vi "SpecAn Marker Peak Read.vi"(0 "VISA In":refnum<visa-resource-name>="N9030A", 5 "Error In":errorcluster={"status"=FALSE, "code"=1073676294, "source"="VISA Read in RS232 Send.vi->Utility Com Write.vi->CG UUT Attenuator Set.vi->CG RF Cal_00.vi"}, 7 "Active Marker":i32(ring)=1 items=["Marker1"=1, "Marker2"=2, "Marker3"=3, "Marker4"=4, "Marker5"=5, "Marker6"=6, "Marker7"=7, "Marker8"=8, "Marker9"=9, "Marker10"=10, "Marker11"=11, "Marker12"=12]) -> (10 "Freq (Hz)":dbl=599400000.0 format="%#_6p", 12 "Amplitude (dBm)":dbl=-83.196 format="%#_6p", 14 "VISA Out":refnum<visa-resource-name>="N9030A", 19 "Error Out":errorcluster={"status"=FALSE, "code"=1073676294, "source"="VISA Read in RS232 Send.vi->Utility Com Write.vi->CG UUT Attenuator Set.vi->CG RF Cal_00.vi"})   [LabVIEW 2015]
uses:
  Controls/FGV Action SpecAn Model.ctl
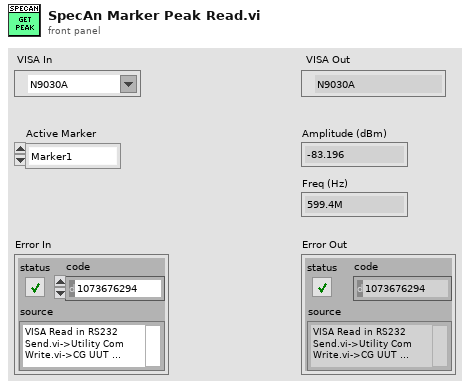
[diagram p1: front panel]
types:
  T1 = typedef "FGV Action SpecAn Model.ctl" = enum16{"Get", "Set"}
  T2 = typedef "SpecAn Model.ctl" = enum16{"E4440", "N9030"}
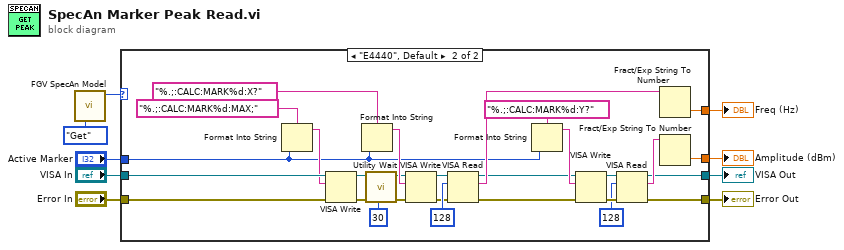
[diagram p0: block diagram]
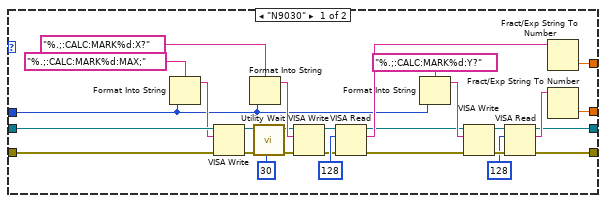
[diagram p2: hidden frame]
diagram:
  n1 = call "FGV SpecAn Model.vi"("Action"=FGV_Action_SpecAn_Model."Get") -> ("SA Model"=w1:T2)  [unwired: 6 in, 1 out]
  n2 = case shown="\"E4440\", Default" w1 {
    tunnel: "VISA In" -> [w34 w61]
    tunnel: "Error In" -> [w33 w60]
    tunnel: [w32 w59] -> w7
    tunnel: [w23 w50] -> w6
    tunnel: "Active Marker" -> [w16 w43]
    tunnel: [w14 w41] -> w4
    tunnel: [w13 w40] -> w3
    frame "N9030" {
      n3 = Format Into String(format string="%.;:CALC:MARK%d:MAX;" ("multi-line string"), w16) -> (resulting string=w31:string)  [unwired: 2 in, 1 out]
      n4 = VISA Write(VISA resource name=w34, write buffer=w31, error in (no error)=w33) -> (VISA resource name out=w28:refnum<visa-resource-name>, error out=w35:errorcluster)  [unwired: 1 out]
      n5 = Format Into String(format string="%.;:CALC:MARK%d:X?" ("multi-line string"), w16) -> (resulting string=w30:string)  [unwired: 2 in, 1 out]
      n6 = call "Utility Wait.vi"("Error In"=w35, "Wait (ms)"=u32 30) -> ("Error Out"=w29:errorcluster)  [unwired: 17 in]
      n7 = VISA Write(VISA resource name=w28, write buffer=w30, error in (no error)=w29) -> (VISA resource name out=w25:refnum<visa-resource-name>, error out=w24:errorcluster)  [unwired: 1 out]
      n8 = VISA Read(VISA resource name=w25, byte count=u32 128, error in (no error)=w24) -> (VISA resource name out=w12:refnum<visa-resource-name>, read buffer=w27:string, error out=w11:errorcluster)  [unwired: 1 out]
      n9 = Format Into String(format string="%.;:CALC:MARK%d:Y?", w16) -> (resulting string=w17:string)  [unwired: 2 in, 1 out]
      n10 = VISA Write(VISA resource name=w12, write buffer=w17, error in (no error)=w11) -> (VISA resource name out=w19:refnum<visa-resource-name>, error out=w20:errorcluster)  [unwired: 1 out]
      n11 = VISA Read(VISA resource name=w19, byte count=u32 128, error in (no error)=w20) -> (VISA resource name out=w14:refnum<visa-resource-name>, read buffer=w15:string, error out=w13:errorcluster)  [unwired: 1 out]
      n12 = Fract/Exp String To Number(string=w27) -> (number=w23:dbl)  [unwired: 3 in, 1 out]
      n13 = Fract/Exp String To Number(string=w15) -> (number=w32:dbl)  [unwired: 3 in, 1 out]
    }
    frame "E4440", Default {
      n14 = Format Into String(format string="%.;:CALC:MARK%d:MAX;" ("multi-line string"), w43) -> (resulting string=w58:string)  [unwired: 2 in, 1 out]
      n15 = VISA Write(VISA resource name=w61, write buffer=w58, error in (no error)=w60) -> (VISA resource name out=w55:refnum<visa-resource-name>, error out=w62:errorcluster)  [unwired: 1 out]
      n16 = Format Into String(format string="%.;:CALC:MARK%d:X?" ("multi-line string"), w43) -> (resulting string=w57:string)  [unwired: 2 in, 1 out]
      n17 = call "Utility Wait.vi"("Error In"=w62, "Wait (ms)"=u32 30) -> ("Error Out"=w56:errorcluster)  [unwired: 17 in]
      n18 = VISA Write(VISA resource name=w55, write buffer=w57, error in (no error)=w56) -> (VISA resource name out=w52:refnum<visa-resource-name>, error out=w51:errorcluster)  [unwired: 1 out]
      n19 = VISA Read(VISA resource name=w52, byte count=u32 128, error in (no error)=w51) -> (VISA resource name out=w39:refnum<visa-resource-name>, read buffer=w54:string, error out=w38:errorcluster)  [unwired: 1 out]
      n20 = Format Into String(format string="%.;:CALC:MARK%d:Y?", w43) -> (resulting string=w44:string)  [unwired: 2 in, 1 out]
      n21 = VISA Write(VISA resource name=w39, write buffer=w44, error in (no error)=w38) -> (VISA resource name out=w46:refnum<visa-resource-name>, error out=w47:errorcluster)  [unwired: 1 out]
      n22 = VISA Read(VISA resource name=w46, byte count=u32 128, error in (no error)=w47) -> (VISA resource name out=w41:refnum<visa-resource-name>, read buffer=w42:string, error out=w40:errorcluster)  [unwired: 1 out]
      n23 = Fract/Exp String To Number(string=w54) -> (number=w50:dbl)  [unwired: 3 in, 1 out]
      n24 = Fract/Exp String To Number(string=w42) -> (number=w59:dbl)  [unwired: 3 in, 1 out]
    }
  }
  "Error Out" <- w3
  "VISA Out" <- w4
  "Amplitude (dBm)" <- w7
  "Freq (Hz)" <- w6
